vi "OP500ZP_FDT_V2.vi"(8 "errin":errorcluster, 9 "TempUsine":dbl) -> (0 "errout":errorcluster, 2 "Log":string, 3 "is OK?":bool, 4 "ToBDD":T1)   [LabVIEW 2020]
uses:
  VG/Ubatt.vi
  VG/PackType.vi
  VG/IS30%.vi
  OP500ZP_VGConf.vi
panel:
  out "PASS/FAIL?":string
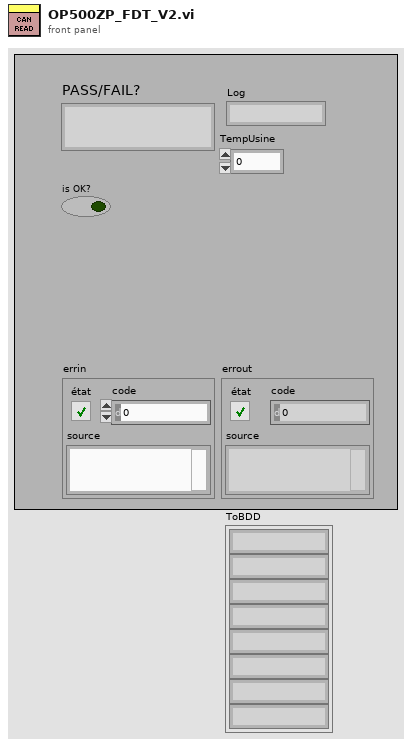
[diagram p1: front panel]
types:
  T1 = cluster{string, string, string, string, string, string, string, string}
  T2 = cluster{"F400 Battery Charge Type":string, "F400 Battery State Request":string, "F400 Ext Insulation Test Control":string, "F400 Int Insulation Test Control":string, "F400 Vehicle Speed":i32, "F400 Ambiant Temperature":i32, "F400 Charger Available Power":i32, "F400 Count":i32, "F106 Keep Active request":string, "F106 Battery State":string, "F106 Operating Status":string, "F106 Battery SOC":dbl, "F106 Battery SOH":dbl, "F106 Ext Insulation Test Status":string, "F106 Int Insulation Test Status":string, "F106 Power Distribution Status":string, "F106 Power Switch Off Delay":i32, "F106 Power Switch Off Request":string, "F106 Count":i32, "F101 Battery Voltage":u32, "F101 Battery Current":dbl, "F101 Max Charge Current":u32, "F101 Max Discharge Current":u32, "F101 Max Discharge Current Temp Limit":string, "F101 Max Discharge Current SOC Limit":string, "F101 Max Charge Current Temp Limit":string, "F101 Max Charge Current SOC Limit":string, "F101 Deliverable Energy":dbl, "F101 Count":u32, "F102 Cell Average Voltage":u32, "F102 Cell Min Voltage":u32, "F102 Cell Max Voltage":u32, "F103 Cell Average Temp":i32, "F103 Cell Min Temp":i32, "F102 Count":u32, "F103 SumOfInternalResistanceT":i32, "F100 Charge Voltage Setpoint":i32, "F100 Charge Current Setpoint":dbl, "F100 Equilization Status":bool, "F100 Charge Competed":bool, "F100 Count":i32, "F107 Outlet Water Temp Request":i32, "F107 Outlet Water Temp Status":i32, "F107 Flow Rate Request":i32, "F107 Inlet Water Temp":i32, "F107 Ambiant Temperature 2":i32, "F105 Max Power Charge Continuous":i32, "F105 Max Power Charge Long Prediction":i32, "F105 Max Power Charge Short Prediction":i32, "F105 Max Current Charge Continuous":i32, "F105 Max Current Charge Short Prediction":i32, "F105 Count ":i32, "F104 Max Power Discharge Continuous":i32, "F104 Max Power Discharge Long Prediction":i32, "F104 Max Power Discharge Short Prediction":i32, "F104 Max Current Discharge Continuous":i32, "F104 Max Current Discharge Short Prediction":i32, "F104 Count ":i32, "F103 Count":i32, "F103 Cell Max Temp":i32, "F103 Max Current Discharge Long Prediction":i32, "F103 Max Current Charge Long Prediction":i32, "F107 Count":i32, "F103 OCV":i32, "F109 DTC":i32}
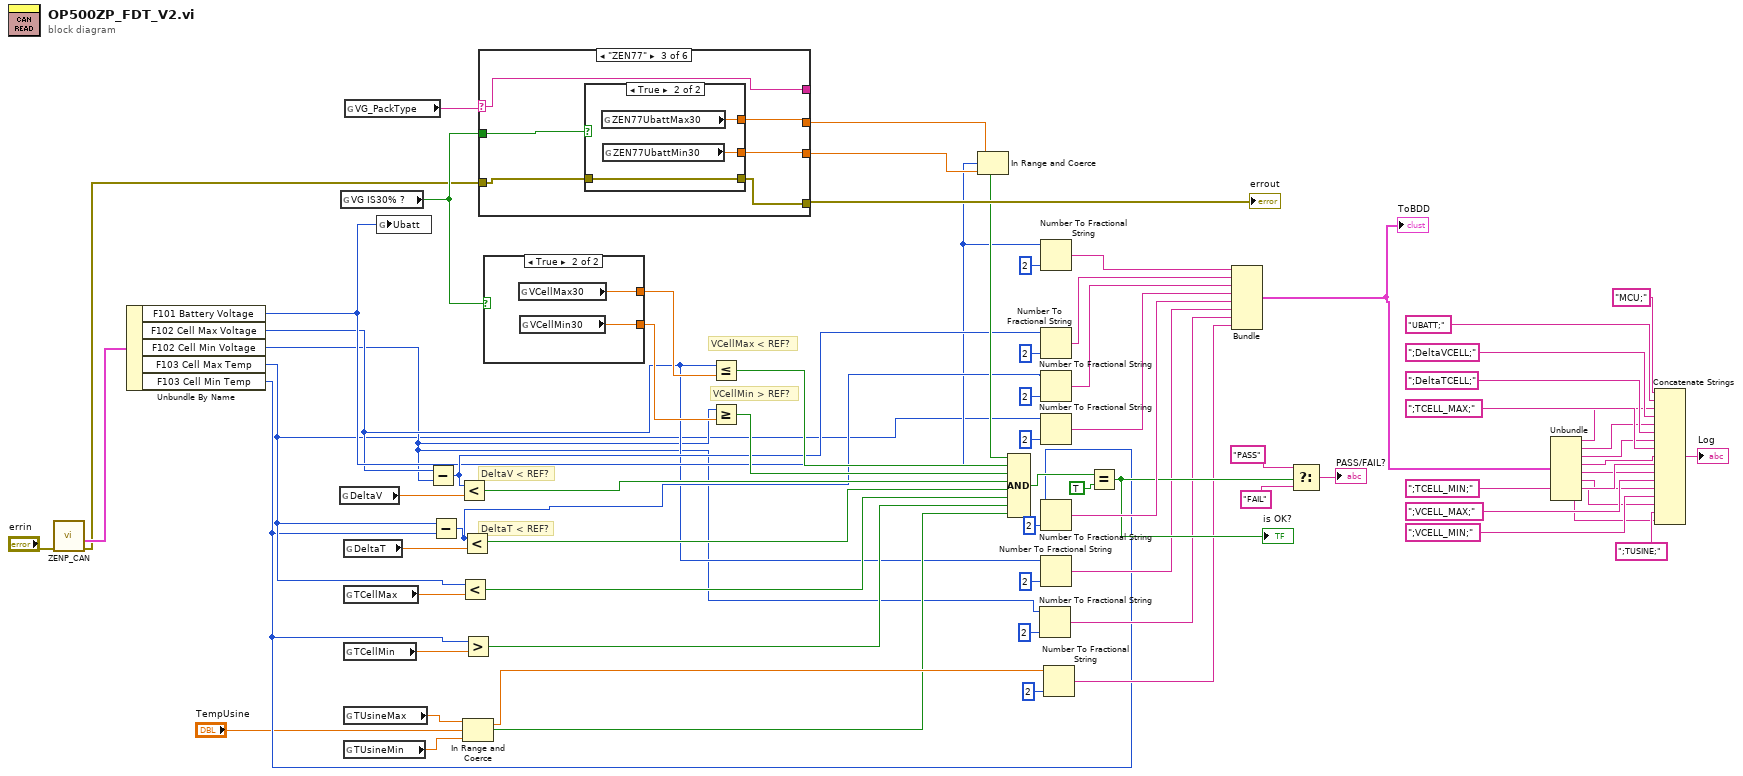
[diagram p0: block diagram]
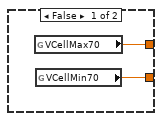
[diagram p2: hidden frame]
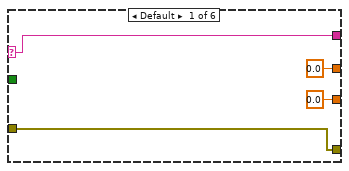
[diagram p3: hidden frame]
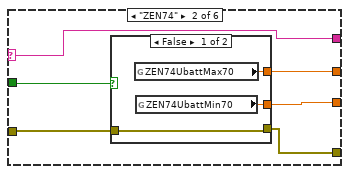
[diagram p4: hidden frame]
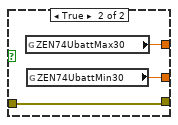
[diagram p5: hidden frame]
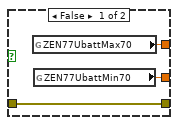
[diagram p6: hidden frame]
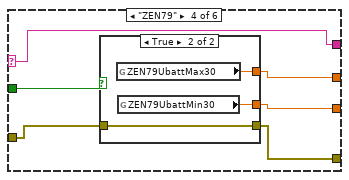
[diagram p7: hidden frame]
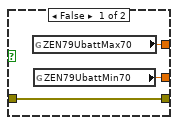
[diagram p8: hidden frame]
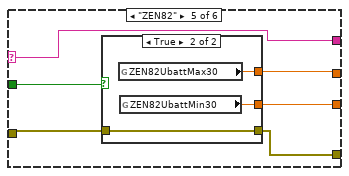
[diagram p9: hidden frame]
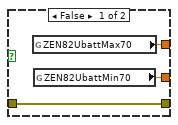
[diagram p10: hidden frame]
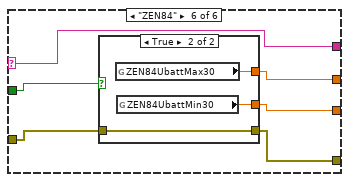
[diagram p11: hidden frame]
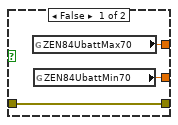
[diagram p12: hidden frame]
diagram:
  # "DeltaT < REF?"
  # "DeltaV < REF?"
  # "VCellMin > REF?"
  # "VCellMax < REF?"
  n1 = call <userlib>:"ZENP_CAN.vi"("errin"="errin") -> ("errout"=w7:errorcluster, "cluster de sortie"=w9:T2)  [unwired: 7 in, 1 out]
  n2 = Unbundle By Name(w9) -> ("F101 Battery Voltage"=w8:u32, "F102 Cell Max Voltage"=w6:u32, "F102 Cell Min Voltage"=w5:u32, "F103 Cell Max Temp"=w4:i32, "F103 Cell Min Temp"=w3:i32)
  n3 = global read "OP500ZP_VGConf.vi" "DeltaV"() -> (w59:dbl)
  n4 = global read "IS30%.vi" "VG IS30% ?"() -> (w57:bool)
  n5 = global read "OP500ZP_VGConf.vi" "DeltaT"() -> (w58:dbl)
  n6 = global read "OP500ZP_VGConf.vi" "TCellMax"() -> (w49:dbl)
  n7 = global read "OP500ZP_VGConf.vi" "TCellMin"() -> (w50:dbl)
  n8 = global read "OP500ZP_VGConf.vi" "TUsineMax"() -> (w41:dbl)
  n9 = global read "OP500ZP_VGConf.vi" "TUsineMin"() -> (w40:dbl)
  n10 = global read "PackType.vi" "VG_PackType"() -> (w74:string)
  n11 = global write "Ubatt.vi" "Ubatt"(w8) -> ()
  n12 = Subtract(x=w6, y=w5) -> (x-y=w46:u32)
  n13 = Subtract(x=w4, y=w3) -> (x-y=w45:i32)
  n14 = Less?(x=w46, y=w59) -> (x < y?=w54:bool)
  n15 = Less?(x=w4, y=w49) -> (x < y?=w48:bool)
  n16 = Less?(x=w45, y=w58) -> (x < y?=w55:bool)
  n17 = Greater?(x=w3, y=w50) -> (0:w47:bool)
  n18 = In Range and Coerce(upper limit=w41, x="TempUsine", lower limit=w40) -> (coerced(x)=w39:dbl, In Range?=w38:bool)
  n19 = case shown="\"ZEN77\"" w74 {
    selector: w74 -> [w78 w81 w93 w105 w117 w129]
    tunnel: [0.0 ("ZEN84UbattMax30") w84 w96 w108 w120 w132] -> w60
    tunnel: [0.0 ("ZEN84UbattMin30") w83 w95 w107 w119 w131] -> w61
    tunnel: w57 -> [_ w82 w94 w106 w118 w130]
    tunnel: [w78 w81 w93 w105 w117 w129] -> _
    tunnel: w7 -> [w77 w80 w92 w104 w116 w128]
    tunnel: [w77 w79 w91 w103 w115 w127] -> w73
    frame Default {
    }
    frame "ZEN74" {
      n20 = case shown="False" w82 {
        tunnel: [w87 w90] -> w84
        tunnel: [w86 w89] -> w83
        tunnel: [w85 w88] -> w79
        tunnel: w80 -> [w85 w88]
        frame False {
          n21 = global read "OP500ZP_VGConf.vi" "ZEN74UbattMax70"() -> (w87:dbl)
          n22 = global read "OP500ZP_VGConf.vi" "ZEN74UbattMin70"() -> (w86:dbl)
        }
        frame True {
          n23 = global read "OP500ZP_VGConf.vi" "ZEN74UbattMax30"() -> (w90:dbl)
          n24 = global read "OP500ZP_VGConf.vi" "ZEN74UbattMin30"() -> (w89:dbl)
        }
      }
    }
    frame "ZEN77" {
      n25 = case shown="True" w94 {
        tunnel: [w99 w102] -> w96
        tunnel: [w98 w101] -> w95
        tunnel: w92 -> [w97 w100]
        tunnel: [w97 w100] -> w91
        frame False {
          n26 = global read "OP500ZP_VGConf.vi" "ZEN77UbattMax70"() -> (w99:dbl)
          n27 = global read "OP500ZP_VGConf.vi" "ZEN77UbattMin70"() -> (w98:dbl)
        }
        frame True {
          n28 = global read "OP500ZP_VGConf.vi" "ZEN77UbattMax30"() -> (w102:dbl)
          n29 = global read "OP500ZP_VGConf.vi" "ZEN77UbattMin30"() -> (w101:dbl)
        }
      }
    }
    frame "ZEN79" {
      n30 = case shown="True" w106 {
        tunnel: [w111 w114] -> w108
        tunnel: [w110 w113] -> w107
        tunnel: w104 -> [w109 w112]
        tunnel: [w109 w112] -> w103
        frame False {
          n31 = global read "OP500ZP_VGConf.vi" "ZEN79UbattMax70"() -> (w111:dbl)
          n32 = global read "OP500ZP_VGConf.vi" "ZEN79UbattMin70"() -> (w110:dbl)
        }
        frame True {
          n33 = global read "OP500ZP_VGConf.vi" "ZEN79UbattMax30"() -> (w114:dbl)
          n34 = global read "OP500ZP_VGConf.vi" "ZEN79UbattMin30"() -> (w113:dbl)
        }
      }
    }
    frame "ZEN82" {
      n35 = case shown="True" w118 {
        tunnel: [w123 w126] -> w120
        tunnel: [w122 w125] -> w119
        tunnel: w116 -> [w121 w124]
        tunnel: [w121 w124] -> w115
        frame False {
          n36 = global read "OP500ZP_VGConf.vi" "ZEN82UbattMax70"() -> (w123:dbl)
          n37 = global read "OP500ZP_VGConf.vi" "ZEN82UbattMin70"() -> (w122:dbl)
        }
        frame True {
          n38 = global read "OP500ZP_VGConf.vi" "ZEN82UbattMax30"() -> (w126:dbl)
          n39 = global read "OP500ZP_VGConf.vi" "ZEN82UbattMin30"() -> (w125:dbl)
        }
      }
    }
    frame "ZEN84" {
      n40 = case shown="True" w130 {
        tunnel: [w135 w138] -> w132
        tunnel: [w134 w137] -> w131
        tunnel: w128 -> [w133 w136]
        tunnel: [w133 w136] -> w127
        frame False {
          n41 = global read "OP500ZP_VGConf.vi" "ZEN84UbattMax70"() -> (w135:dbl)
          n42 = global read "OP500ZP_VGConf.vi" "ZEN84UbattMin70"() -> (w134:dbl)
        }
        frame True {
          n43 = global read "OP500ZP_VGConf.vi" "ZEN84UbattMax30"() -> (w138:dbl)
          n44 = global read "OP500ZP_VGConf.vi" "ZEN84UbattMin30"() -> (w137:dbl)
        }
      }
    }
  }
  "errout" <- w73
  n45 = case shown="True" w57 {
    tunnel: [w140 w142] -> w56
    tunnel: [w139 w141] -> w43
    frame False {
      n46 = global read "OP500ZP_VGConf.vi" "VCellMax70"() -> (w140:dbl)
      n47 = global read "OP500ZP_VGConf.vi" "VCellMin70"() -> (w139:dbl)
    }
    frame True {
      n48 = global read "OP500ZP_VGConf.vi" "VCellMax30"() -> (w142:dbl)
      n49 = global read "OP500ZP_VGConf.vi" "VCellMin30"() -> (w141:dbl)
    }
  }
  n50 = Less Or Equal?(x=w6, y=w56) -> (x <= y?=w52:bool)
  n51 = Greater Or Equal?(x=w5, y=w43) -> (x >= y?=w53:bool)
  n52 = In Range and Coerce(upper limit=w60, x=w8, lower limit=w61) -> (In Range?=w51:bool)  [unwired: 1 out]
  n53 = Compound Arithmetic op=AND ("Opérateur arithmétique")(w51, w52, w53, w54, w55, w48, w47, w38) -> (w67:bool)
  n54 = Number To Fractional String(number=w5, precision (6)=i16 2 ("précision (6)")) -> (F-format string=w42:string)  [unwired: 2 in]
  n55 = Number To Fractional String(number=w8, precision (6)=i16 2 ("précision (6)")) -> (F-format string=w72:string)  [unwired: 2 in]
  n56 = Number To Fractional String(number=w46, precision (6)=i16 2 ("précision (6)")) -> (F-format string=w71:string)  [unwired: 2 in]
  n57 = Number To Fractional String(number=w45, precision (6)=i16 2 ("précision (6)")) -> (F-format string=w70:string)  [unwired: 2 in]
  n58 = Number To Fractional String(number=w4, precision (6)=i16 2 ("précision (6)")) -> (F-format string=w69:string)  [unwired: 2 in]
  n59 = Number To Fractional String(number=w3, precision (6)=i16 2 ("précision (6)")) -> (F-format string=w68:string)  [unwired: 2 in]
  n60 = Number To Fractional String(number=w6, precision (6)=i16 2 ("précision (6)")) -> (F-format string=w44:string)  [unwired: 2 in]
  n61 = Number To Fractional String(number=w39, precision (6)=i16 2 ("précision (6)")) -> (F-format string=w37:string)  [unwired: 2 in]
  n62 = Equal?(x=w67, y=TRUE) -> (x = y?=w63:bool)
  "is OK?" <- w63
  n63 = Bundle(w72, w71, w70, w69, w68, w44, w42, w37) -> (w11:T1)  [unwired: 1 in]
  "ToBDD" <- w11
  n64 = Select ("Sélectionner")(t="PASS", s=w63, f="FAIL") -> (s? t:f=→"PASS/FAIL?":string)
  n65 = Unbundle(w11) -> (w21:string, w20:string, w19:string, w18:string, w17:string, w16:string, w15:string, w12:string)
  n66 = Concatenate Strings("MCU;" ("chaîne"), "UBATT;", w21, ";DeltaVCELL;", w20, ";DeltaTCELL;", w19, ";TCELL_MAX;", w18, ";TCELL_MIN;", w17, ";VCELL_MAX;", w16, ";VCELL_MIN;", w15, ";TUSINE;" ("chaîne"), w12) -> (→"Log":string)
